vi "Agilent Custom Gains.vi"(8 "Error In":errorcluster, 10 "Analog Channels-List":string, 11 "TC Channels-List":string) -> (0 "Error Out":errorcluster, 1 "Clean TC Scan List":string, 2 "Clean Analog Scan List":string, 3 "Total Clean Scan List":string)   [LabVIEW 2018]
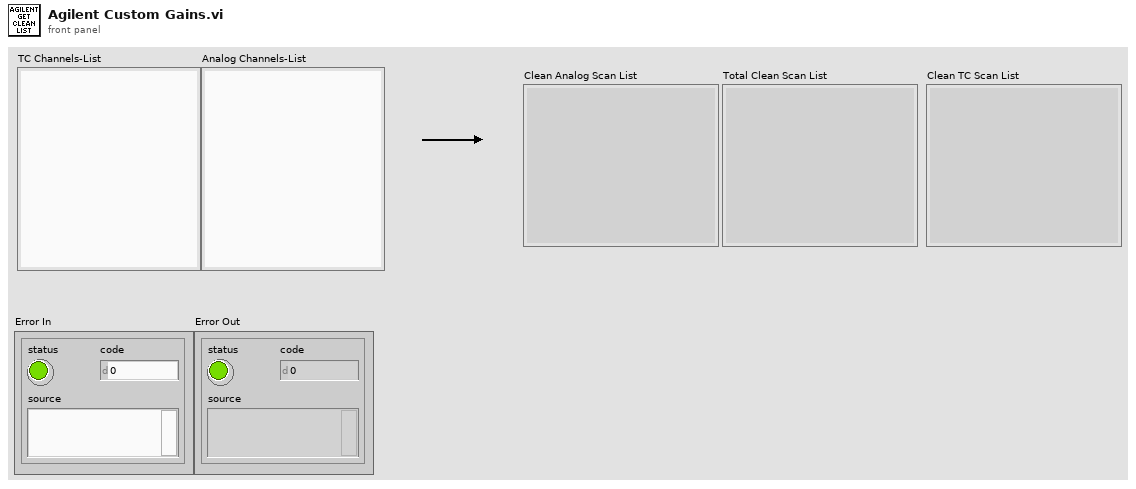
[diagram p1: front panel]
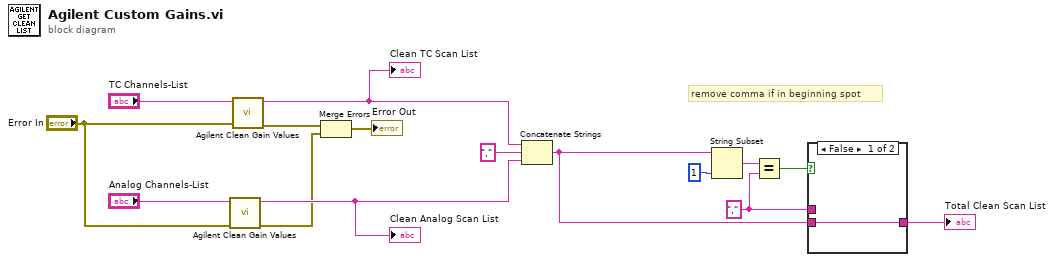
[diagram p0: block diagram]
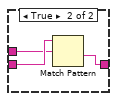
[diagram p2: hidden frame]
diagram:
  w12 = "," ("y")
  # "remove comma if in beginning spot"
  n1 = call "Agilent Clean Gain Values.vi"("Error In"="Error In", "Analog Channels-List"="Analog Channels-List") -> ("Error Out"=w3:errorcluster, "String"=w15:string)  [unwired: 8 in]
  "Clean Analog Scan List" <- w15
  n2 = call "Agilent Clean Gain Values.vi"("Error In"="Error In", "Analog Channels-List"="TC Channels-List") -> ("Error Out"=w4:errorcluster, "String"=w1:string)  [unwired: 8 in]
  "Clean TC Scan List" <- w1
  n3 = Merge Errors(w4, w3) -> (→"Error Out":errorcluster)
  n4 = Concatenate Strings(w1, "," ("string"), w15) -> (w11:string)
  n5 = String Subset(string=w11, length (rest)=1 ("length (rest)")) -> (substring=w9:string)  [unwired: 1 in]
  n6 = Equal?(x=w9, y=w12) -> (x = y?=w10:bool)
  n7 = case shown="False" w10 {
    tunnel: w11 -> [w16 w19]
    tunnel: w12 -> [_ w18]
    tunnel: [w16 w17] -> w13
    frame False {
    }
    frame True {
      n8 = Match Pattern(string=w19, regular expression=w18) -> (after substring=w17:string)  [unwired: 1 in, 3 out]
    }
  }
  "Total Clean Scan List" <- w13
